vi "test Get Distance From AnchorDistanceArray By TagID Correct.vi"(8 "error in (no error)":errorcluster, 11 "TestCase in":refnum<class "Utility VIs tests.lvclass">) -> (0 "error out":errorcluster, 3 "TestCase out":refnum<class "Utility VIs tests.lvclass">)   [LabVIEW 2014, in "Utility VIs tests.lvclass"]
uses:
  Utility VIs tests.lvclass
  SPLAT/Tag.lvclass
  <vilib>/addons/_JKI Toolkits/VI Tester/TestCase.llb/TestCase.lvclass
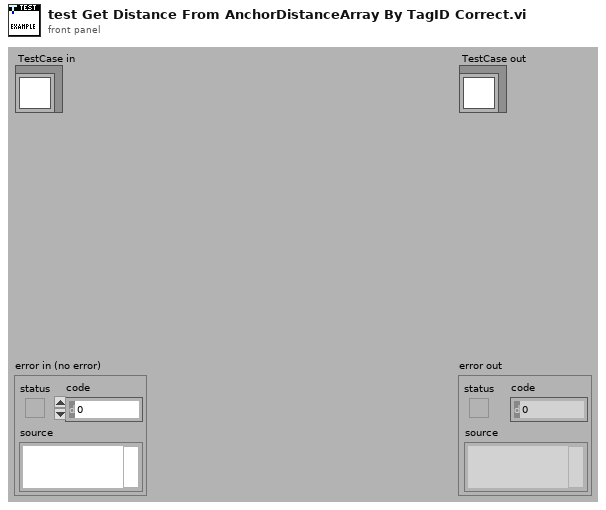
[diagram p1: front panel]
types:
  T1 = cluster{"Tag.lvclass":refnum<class "Tag.lvclass">, "Distance":dbl}[]
  T2 = cluster{"Tag Out":refnum<class "Tag.lvclass">, dbl}
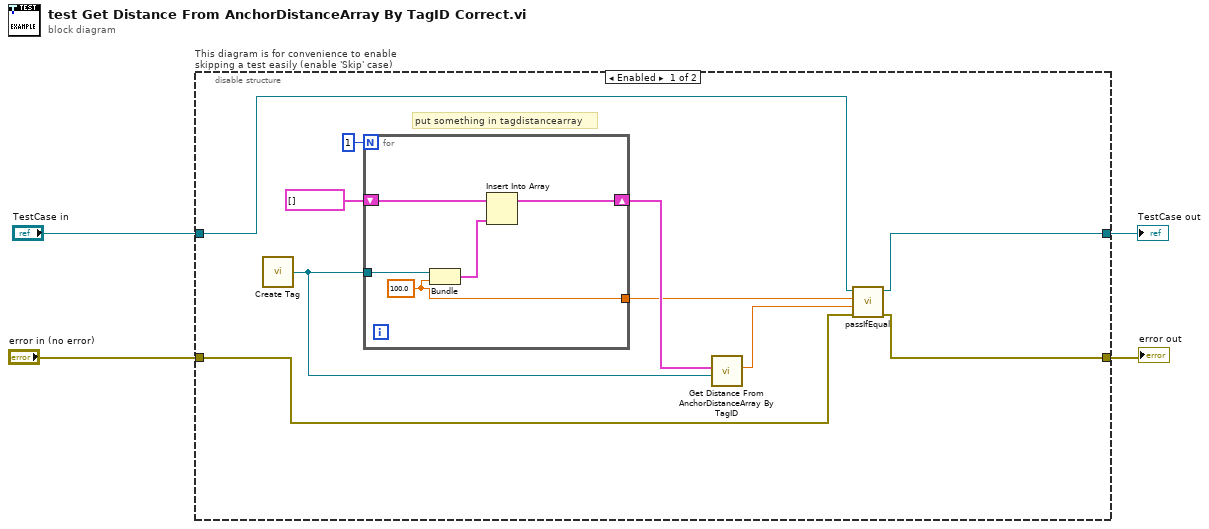
[diagram p0: block diagram]
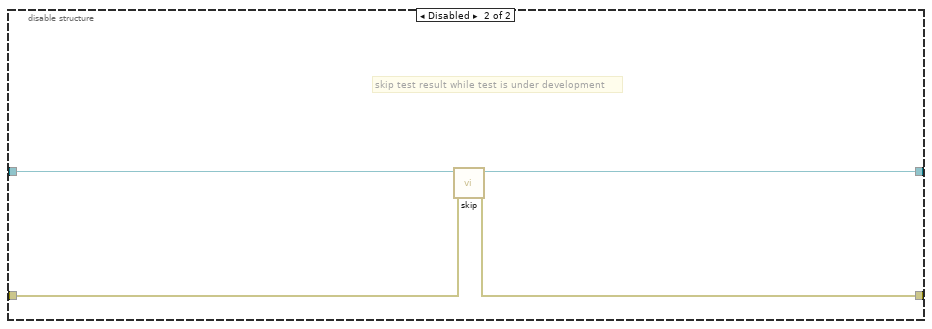
[diagram p2: hidden frame]
diagram:
  n1 = disable-structure "This diagram is for convenience to enable skipping a test easily (enable 'Skip' case)" shown="Enabled" {
    disable-tunnel: "TestCase in" -> [w8 w23]
    disable-tunnel: [w7 w21] -> w1
    disable-tunnel: [w9 w22] -> w3
    disable-tunnel: "error in (no error)" -> [w10 w20]
    frame Enabled {
      # "put something in tagdistancearray"
      n2 = call "Create Tag.vi"() -> ("Tag Out"=w13:refnum<class "Tag.lvclass">)  [unwired: 3 in]
      n3 = for {
        N: 1 -> [_]
        shift-right: [w16] -> w12
        shift-left: T1 [] ("Input TagDistanceArray") -> [w19]
        tunnel: w13 -> [w17]
        tunnel: [w15] -> w5
        w15 = 100.0
        n4 = Bundle("Tag Out"=w17, w15) -> (w18:T2)  [unwired: 1 in]
        n5 = Insert Into Array(array=w19, new element=w18) -> (w16:T1)  [unwired: 1 in]
      }
      n6 = call "Get Distance From AnchorDistanceArray By TagID.vi"("Tag.lvclass"=w13, "Input TagDistanceArray"=w12) -> ("Distance"=w6:dbl)  [unwired: 9 in]
      n7 = call-dynamic "passIfEqual.vi"("error in (no error)"=w10, "y"=w6, "x"=w5, "TestCase in"=w8) -> ("error out"=w9:errorcluster, "TestCase out"=w7:refnum<class "Utility VIs tests.lvclass">)  [unwired: 6 in]
    }
    frame Disabled {
      # "skip test result while test is under development"
      n8 = call <vilib>:"skip.vi"("error in (no error)"=w20, "TestCase in"=w23) -> ("error out"=w22:errorcluster, "TestCase out"=w21:refnum<class "Utility VIs tests.lvclass">)  [unwired: 8 in]
    }
  }
  "error out" <- w3
  "TestCase out" <- w1
